vi "PoseAndTargeting.vi"(0 "disabledRunning":bool, 1 "moduleDriveVelocityTicksPer100ms":T1, 2 "moduleDrivePositionTicks":T2, 5 "Initial X Position (m)":dbl, 9 "Initial Y Position (m)":dbl, 11 "autoArray":dbl[][](array[numeric])) -> (6 "X Position (m)":dbl, 10 "Y Position (m)":dbl)   [LabVIEW 2020]
doc: "This VI manages the robot's pose and targetting information. Data from the IMU, swerve drive encoders, swerve azimuth encoders, LimeLight, and LIDAR are fused together to estimate these values. Supports pose resets on boot, from the Autonomous Sequencer, and on command from the FRC 4265 Dashboard."
uses:
  <vilib>/Rock Robotics/WPI/ThirdParty/Phoenix-LabVIEW/Pigeon IMU/CTRE_PigeonIMU_TareType.ctl
  Team Code/Robot Global Data.vi
panel:
  out "swerveGroundSpeed":dbl
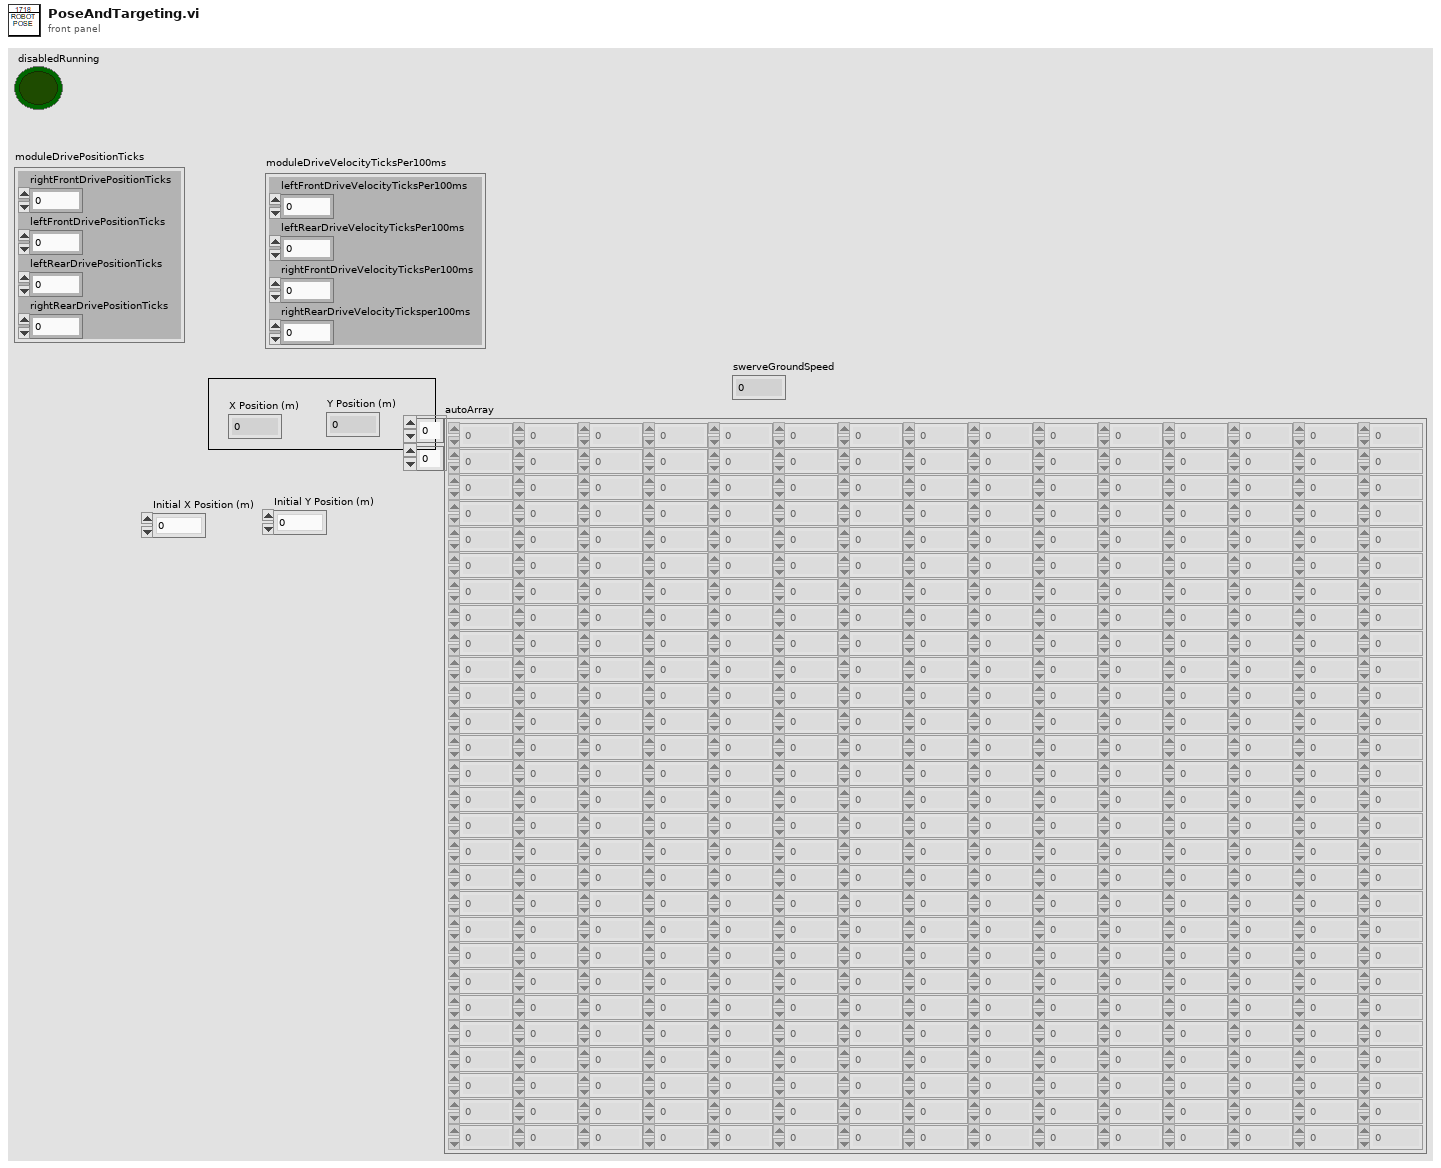
[diagram p1: front panel]
types:
  T1 = cluster{"leftFrontDriveVelocityTicksPer100ms":dbl, "leftRearDriveVelocityTicksPer100ms":dbl, "rightFrontDriveVelocityTicksPer100ms":dbl, "rightRearDriveVelocityTicksper100ms":dbl}
  T2 = cluster{"rightFrontDrivePositionTicks":dbl, "leftFrontDrivePositionTicks":dbl, "leftRearDrivePositionTicks":dbl, "rightRearDrivePositionTicks":dbl}
  T3 = typedef "Absolute Angle TypeDef.ctl" = cluster{"leftFrontAbsoluteAngle":dbl, "leftRearAbsoluteAngle":dbl, "rightFrontAbsoluteAngle":dbl, "rightRearAbsoluteAngle":dbl}
  T4 = typedef "CTRE_PigeonIMU_TareType.ctl" = u8
  T5 = typedef "CTRE_PigeonIMU_DeviceRef.ctl" = cluster{"DeviceStatus":errorcluster, "Device Number":u8, "Type":T6, "Device ID":u32, "Handle":u64, "UsageFrame":u32, "Library Path":path}
  T6 = typedef "CTRE_PigeonIMU_ConnectionType.ctl" = u32
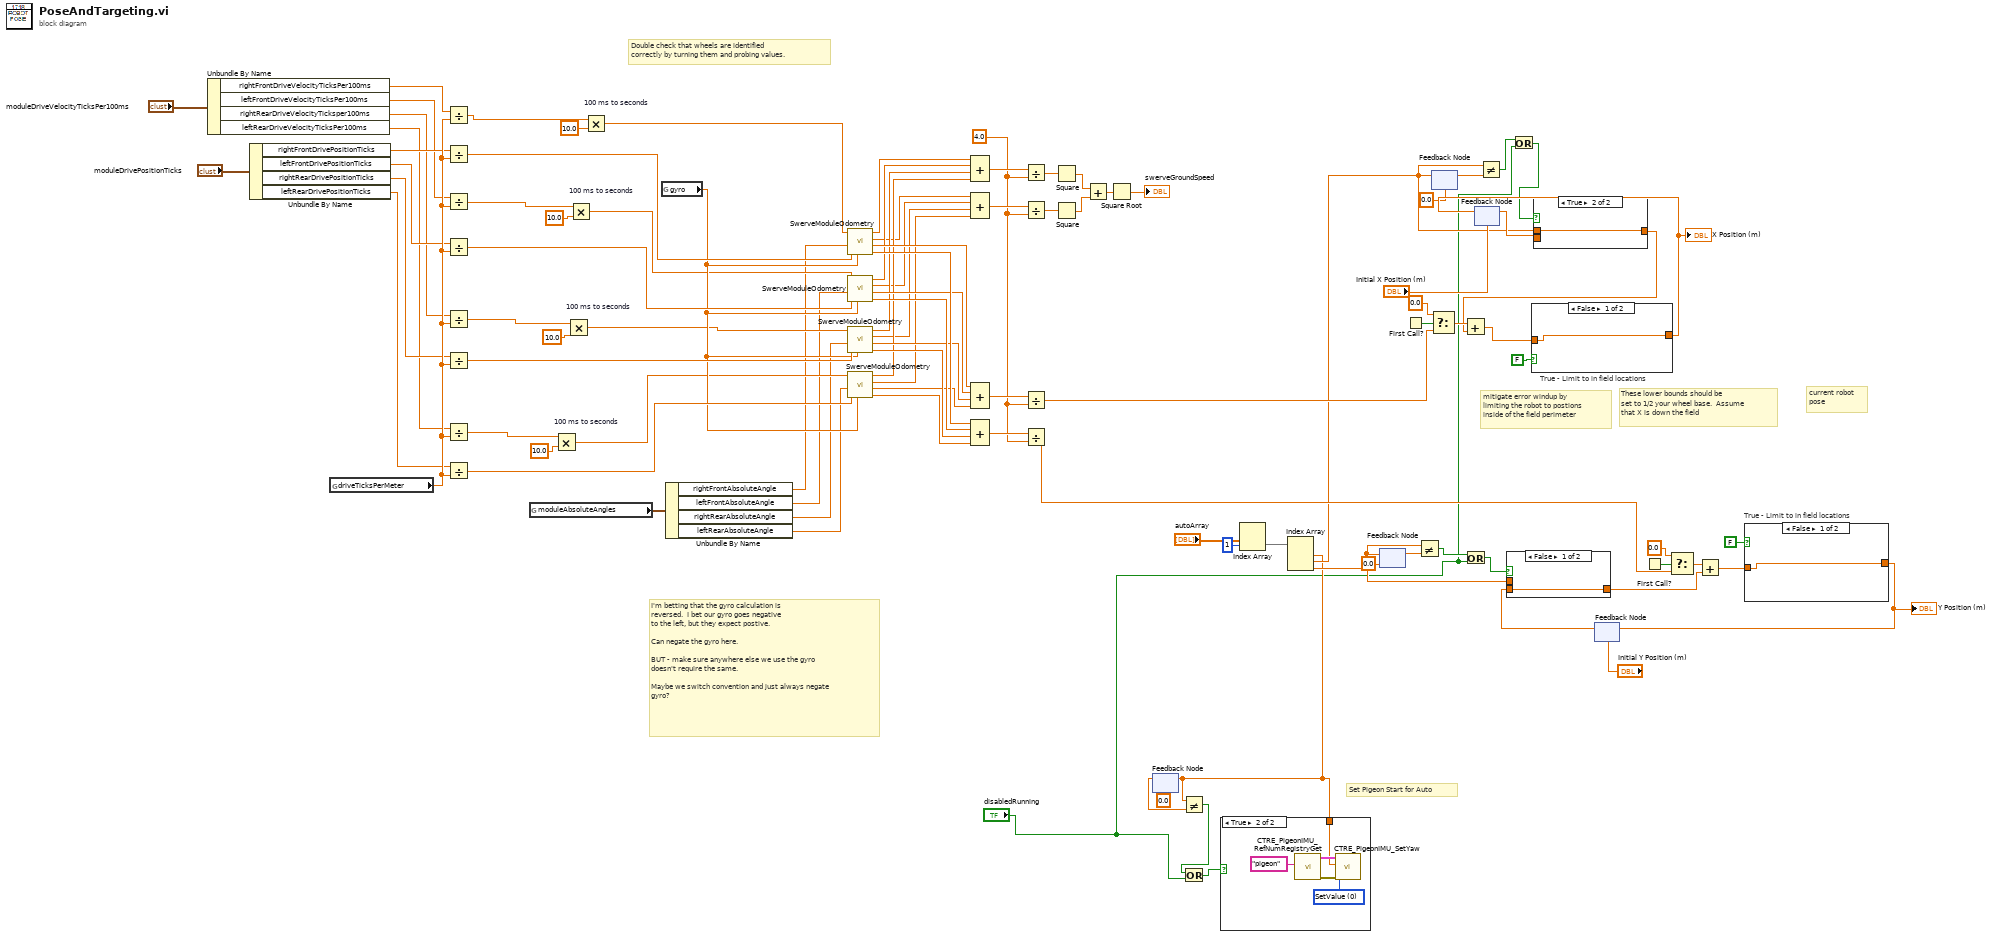
[diagram p0: block diagram]
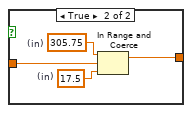
[diagram p5: hidden frame]
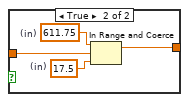
[diagram p6: hidden frame]
diagram:
  w65 = 4.0 ("upper limit")
  # "Set Pigeon Start for Auto"
  # "I'm betting that the gyro calculation is\nreversed.  I bet our gyro goes negative\nto the left, but they expect postive.\n\nCan negate the gyro here.\n\nBUT - make sure anywhere else we use the gyro\ndoesn't require the same.\n\nMaybe we switch convention and just always negate\ngyro?"
  # "Double check that wheels are identified\ncorrectly by turning them and probing values."
  # "These lower bounds should be\nset to 1/2 your wheel base.  Assume\nthat X is down the field"
  # "current robot\npose"
  # "mitigate error windup by\nlimiting the robot to postions\ninside of the field perimeter"
  n1 = Unbundle By Name("moduleDriveVelocityTicksPer100ms") -> ("rightFrontDriveVelocityTicksPer100ms"=w33:dbl, "leftFrontDriveVelocityTicksPer100ms"=w31:dbl, "rightRearDriveVelocityTicksper100ms"=w32:dbl, "leftRearDriveVelocityTicksPer100ms"=w30:dbl)
  n2 = Unbundle By Name("moduleDrivePositionTicks") -> ("rightFrontDrivePositionTicks"=w38:dbl, "leftFrontDrivePositionTicks"=w37:dbl, "rightRearDrivePositionTicks"=w36:dbl, "leftRearDrivePositionTicks"=w35:dbl)
  n3 = global read "Robot Global Data.vi" "driveTicksPerMeter"() -> (w40:dbl)
  n4 = Divide(x=w33, y=w40) -> (x/y=w16:dbl)
  n5 = Divide(x=w38, y=w40) -> (x/y=w58:dbl)
  n6 = Divide(x=w31, y=w40) -> (x/y=w15:dbl)
  n7 = Divide(x=w37, y=w40) -> (x/y=w61:dbl)
  n8 = Divide(x=w32, y=w40) -> (x/y=w14:dbl)
  n9 = Divide(x=w36, y=w40) -> (x/y=w60:dbl)
  n10 = Divide(x=w30, y=w40) -> (x/y=w13:dbl)
  n11 = Divide(x=w35, y=w40) -> (x/y=w59:dbl)
  n12 = global read "Robot Global Data.vi" "moduleAbsoluteAngles"() -> (w45:T3)
  n13 = Multiply "100 ms to seconds"(x=w13, y=10.0) -> (x*y=w50:dbl)
  n14 = Multiply "100 ms to seconds"(x=w14, y=10.0) -> (x*y=w49:dbl)
  n15 = Multiply "100 ms to seconds"(x=w15, y=10.0) -> (x*y=w48:dbl)
  n16 = Multiply "100 ms to seconds"(x=w16, y=10.0) -> (x*y=w54:dbl)
  n17 = global read "Robot Global Data.vi" "gyro"() -> (w57:dbl)
  n18 = Unbundle By Name(w45) -> ("rightFrontAbsoluteAngle"=w44:dbl, "leftFrontAbsoluteAngle"=w43:dbl, "rightRearAbsoluteAngle"=w41:dbl, "leftRearAbsoluteAngle"=w42:dbl)
  n19 = call "SwerveModuleOdometry.vi"("Robot Heading(deg)"=w57, "Wheel Distance (m)"=w58, "Wheel Azimuth (deg)"=w44, "Velocity (m/s)"=w54) -> ("Delta Y (m)"=w94:dbl, "Delta X (m)"=w84:dbl, "Velocity Y (m/s)"=w76:dbl, "Velocity X (m/s)"=w80:dbl)  [unwired: 2 in]
  n20 = call "SwerveModuleOdometry.vi"("Robot Heading(deg)"=w57, "Wheel Distance (m)"=w61, "Wheel Azimuth (deg)"=w43, "Velocity (m/s)"=w48) -> ("Delta Y (m)"=w95:dbl, "Delta X (m)"=w83:dbl, "Velocity Y (m/s)"=w75:dbl, "Velocity X (m/s)"=w79:dbl)  [unwired: 2 in]
  n21 = call "SwerveModuleOdometry.vi"("Robot Heading(deg)"=w57, "Wheel Distance (m)"=w60, "Wheel Azimuth (deg)"=w41, "Velocity (m/s)"=w49) -> ("Delta Y (m)"=w96:dbl, "Delta X (m)"=w82:dbl, "Velocity Y (m/s)"=w74:dbl, "Velocity X (m/s)"=w78:dbl)  [unwired: 2 in]
  n22 = call "SwerveModuleOdometry.vi"("Robot Heading(deg)"=w57, "Wheel Distance (m)"=w59, "Wheel Azimuth (deg)"=w42, "Velocity (m/s)"=w50) -> ("Delta Y (m)"=w97:dbl, "Delta X (m)"=w81:dbl, "Velocity Y (m/s)"=w73:dbl, "Velocity X (m/s)"=w77:dbl)  [unwired: 2 in]
  n23 = Compound Arithmetic op=ADD(w80, w79, w78, w77) -> (w72:dbl)
  n24 = Compound Arithmetic op=ADD(w76, w75, w74, w73) -> (w71:dbl)
  n25 = Compound Arithmetic op=ADD(w84, w83, w82, w81) -> (w99:dbl)
  n26 = Compound Arithmetic op=ADD(w94, w95, w96, w97) -> (w98:dbl)
  n27 = Divide(x=w72, y=w65) -> (x/y=w67:dbl)
  n28 = Divide(x=w71, y=w65) -> (x/y=w66:dbl)
  n29 = Divide(x=w99, y=w65) -> (x/y=w64:dbl)
  n30 = Divide(x=w98, y=w65) -> (x/y=w63:dbl)
  n31 = Square(x=w67) -> (x^2=w69:dbl)
  n32 = Square(x=w66) -> (x^2=w70:dbl)
  n33 = Add(x=w69, y=w70) -> (x+y=w68:dbl)
  n34 = Square Root(x=w68) -> (sqrt(x)=→"swerveGroundSpeed":dbl)
  n35 = feedback #1(0.0 ("Numeric")) -> (w10:dbl)
  n36 = Index Array(array="autoArray", index (row)=1) -> (element=w25:dbl[])  [unwired: 1 in]
  n37 = Index Array(array=w25) -> (element #1=w9:dbl, element #2=w18:dbl, element #3=w21:dbl)  [unwired: 3 in]
  n38 = feedback-in #1(w9) -> ()
  n39 = Not Equal?(x=w9, y=w10) -> (x != y?=w7:bool)
  n40 = Or(x=w7, y="disabledRunning") -> (x .or. y?=w6:bool)
  n41 = case shown="True" w6 {
    tunnel: w9 -> [_ w101]
    frame False {
    }
    frame True {
      w100 = T4 0 items=["SetValue"=0, "AddOffset"=1, "MatchCompass"=2, "SetOffset"=255] ("TareType (SetValue)")
      n42 = call <vilib>:"CTRE_PigeonIMU_RefNumRegistryGet.vi"("refnum name"="pigeon") -> ("error out"=w104:errorcluster, "PigeonIMUDevRef"=w103:T5)  [unwired: 9 in]
      n43 = call <vilib>:"CTRE_PigeonIMU_SetYaw.vi"("error in (no error)"=w104, "TareType (SetValue)"=w100, "Value"=w101, "PigeonIMUDevRef"=w103) -> ()  [unwired: 6 in, 2 out]
    }
  }
  n44 = feedback #2(0.0 ("Numeric")) -> (w22:dbl)
  n45 = feedback-in #2(w21) -> ()
  n46 = First Call?() -> (First Call?: T/F=w92:bool)
  n47 = Not Equal?(x=w21, y=w22) -> (x != y?=w5:bool)
  n48 = Select(t=0.0, s=w92, f=w64) -> (s? t:f=w93:dbl)
  n49 = feedback #3(0.0 ("Numeric")) -> (w20:dbl)
  n50 = feedback-in #3(w18) -> ()
  n51 = Or(x=w5, y="disabledRunning") -> (x .or. y?=w4:bool)
  n52 = feedback #4("Initial X Position (m)") -> (w19:dbl)
  n53 = Not Equal?(x=w18, y=w20) -> (x != y?=w3:bool)
  n54 = Or(x=w3, y="disabledRunning") -> (x .or. y?=w2:bool)
  n55 = case shown="True" w2 {
    tunnel: w19 -> [w105 _]
    tunnel: w18 -> [_ w106]
    tunnel: [w105 w106] -> w17
    frame False {
    }
    frame True {
    }
  }
  n56 = Add(x=w93, y=w17) -> (x+y=w87:dbl)
  n57 = case "True - Limit to in field locations" shown="False" FALSE {
    tunnel: w87 -> [w107 w109]
    tunnel: [w107 w108] -> w85
    frame False {
    }
    frame True {
      w110 = 611.75  # (in)
      w111 = 17.5  # (in)
      n58 = In Range and Coerce(upper limit=w110, x=w109, lower limit=w111) -> (coerced(x)=w108:dbl)  [unwired: 1 out]
    }
  }
  "X Position (m)" <- w85
  n59 = feedback-in #4(w85) -> ()
  n60 = feedback #5("Initial Y Position (m)") -> (w24:dbl)
  n61 = case shown="False" w4 {
    tunnel: w24 -> [w112 _]
    tunnel: [w112 w113] -> w23
    tunnel: w21 -> [_ w113]
    frame False {
    }
    frame True {
    }
  }
  n62 = First Call?() -> (First Call?: T/F=w89:bool)
  n63 = Select(t=0.0, s=w89, f=w63) -> (s? t:f=w90:dbl)
  n64 = Add(x=w90, y=w23) -> (x+y=w86:dbl)
  n65 = case "True - Limit to in field locations" shown="False" FALSE {
    tunnel: w86 -> [w114 w116]
    tunnel: [w114 w115] -> w56
    frame False {
    }
    frame True {
      w117 = 305.75  # (in)
      w118 = 17.5  # (in)
      n66 = In Range and Coerce(upper limit=w117, x=w116, lower limit=w118) -> (coerced(x)=w115:dbl)  [unwired: 1 out]
    }
  }
  "Y Position (m)" <- w56
  n67 = feedback-in #5(w56) -> ()
